vi "VI-Show Library.vi"(0 "Library Path":path, 11 "error in (no error)":errorcluster) -> (15 "error out":errorcluster)   [LabVIEW 2020]
panel:
  in  "LVClassLibrary in":refnum<vi>
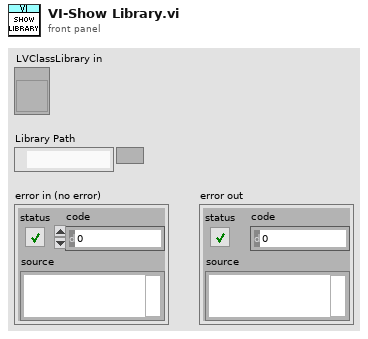
[diagram p1: front panel]
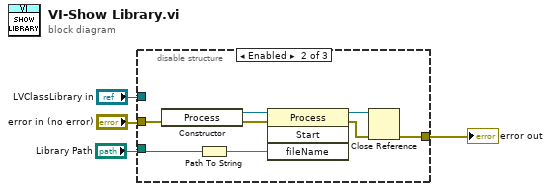
[diagram p0: block diagram]
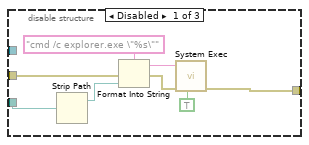
[diagram p2: hidden frame]
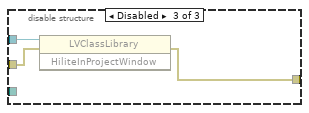
[diagram p3: hidden frame]
diagram:
  n1 = disable-structure shown="Enabled" {
    disable-tunnel: "error in (no error)" -> [w12 w13 w22]
    disable-tunnel: [w11 w14 w21] -> w1
    disable-tunnel: "Library Path" -> [w5 w15 _]
    disable-tunnel: "LVClassLibrary in" -> [_ _ w23]
    frame Disabled {
      n2 = Strip Path(path=w5) -> (stripped path=w6:path)  [unwired: 1 out]
      n3 = Format Into String(format string="cmd /c explorer.exe \"%s\"", error in=w12, w6) -> (resulting string=w9:string, error out=w7:errorcluster)  [unwired: 1 in]
      n4 = call <vilib>:"System Exec.vi"("run minimized? (F)"=TRUE, "error in (no error)"=w7, "command line"=w9) -> ("error out"=w11:errorcluster)  [unwired: 5 in, 3 out]
    }
    frame Enabled {
      n5 = constructor class="Process"(error in=w13) -> (reference out=w17:refnum<k24>, error out=w16:errorcluster)  [unwired: 2 in, 1 out]
      n6 = Path To String(path=w15) -> (string=w20:string)
      n7 = invoke class="Process" method="Start"(reference=w17, error in=w16, "fileName"=w20) -> (reference out=w19:refnum<k24>, error out=w18:errorcluster)  [unwired: 1 in, 2 out]
      n8 = Close Reference(reference=w19, error in (no error)=w18) -> (error out=w14:errorcluster)
    }
    frame Disabled {
      n9 = invoke class="LVClassLibrary" method="HiliteInProjectWindow"(reference=w23, error in=w22) -> (error out=w21:errorcluster)  [unwired: 1 in, 2 out]
    }
  }
  "error out" <- w1
